vi "Wait For Exit.vi"(7 "timeout [ms]":i32=-1, 8 "error in":errorcluster, 11 "pipe in":T1) -> (0 "error out":errorcluster, 2 "exit code":i32, 3 "pipe out":T1)   [LabVIEW 2013, in "LV Process library.lvlib"]
doc: "Calls lv_proc.dll to wait for process exit. Be carefull using this without timeout (default1) because it will hangup until process returnes. It does not terminates the process, it only waits until it finishes."
uses:
  LV Process library.lvlib
  Pipe Handle.ctl
panel:
  out "exited?":bool
  in  "code mem":i32
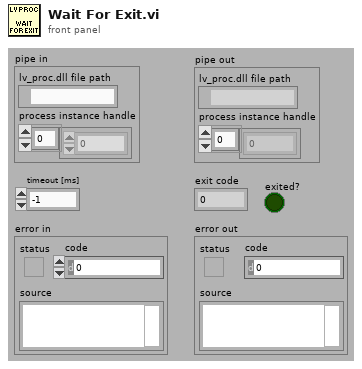
[diagram p1: front panel]
types:
  T1 = typedef "LV Process library.lvlib/Pipe Handle.ctl" = cluster{"lv_proc.dll file path":path, "process instance handle":u32[]}
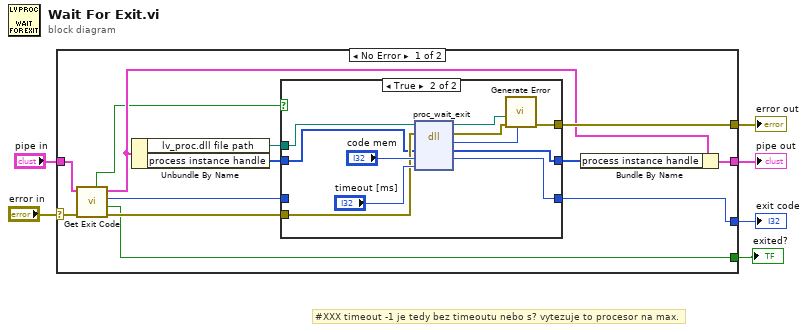
[diagram p0: block diagram]
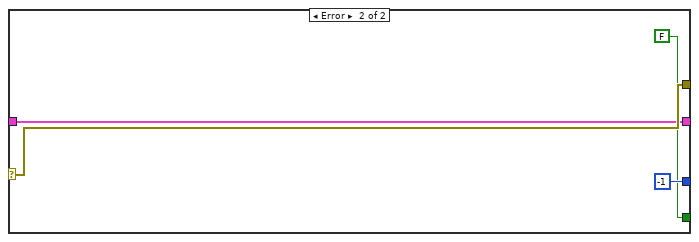
[diagram p3: hidden frame]
diagram:
  # "#XXX timeout -1 je tedy bez timeoutu nebo s? vytezuje to procesor na max."
  n1 = case shown="No Error" "error in" {
    selector: "error in" -> [w8 w37]
    tunnel: [w19 w37] -> w6
    tunnel: [w18 -1 ("code")] -> w5
    tunnel: [w16 w36] -> w4
    tunnel: "pipe in" -> [w14 w36]
    tunnel: [w7 FALSE ("exited?")] -> w1
    frame No Error {
      n2 = call "Get Exit Code.vi"("error in"=w8, "pipe in"=w14) -> ("error out"=w12:errorcluster, "exited?"=w7:bool, "exit code"=w9:i32, "pipe out"=w13:T1, "running?"=w11:bool)  [unwired: 5 in]
      n3 = Unbundle By Name(w13) -> ("lv_proc.dll file path"=w17:path, "process instance handle"=w10:u32[])
      n4 = case shown="True" w11 {
        tunnel: [w22 w23] -> w19
        tunnel: [w20 w31] -> w18
        tunnel: [w21 w26] -> w15
        tunnel: w12 -> [w22 w30]
        tunnel: w10 -> [w21 w29]
        tunnel: w9 -> [w20 _]
        tunnel: w17 -> [_ w28]
        frame False {
        }
        frame True {
          n5 = dll-call lib="lv_proc.dll" fn="proc_wait_exit"(path in=w28, error in=w30, "proc"=w29, "code"="code mem", "timeout [ms]"="timeout [ms]") -> (path out=w25:path, error out=w24:errorcluster, "error"=w27:i32, "proc"=w26:u32[], "code"=w31:i32)  [unwired: 2 in]
          n6 = call "Generate Error.vi"("error code in"=w27, "error in"=w24, "lv_proc.dll path in"=w25) -> ("error out"=w23:errorcluster)  [unwired: 6 in, 1 out]
        }
      }
      n7 = Bundle By Name(cluster=w13, "process instance handle"=w15) -> (w16:T1)
    }
    frame Error {
    }
  }
  "error out" <- w6
  "exit code" <- w5
  "pipe out" <- w4
  "exited?" <- w1
